vi "TEST_L0_SUM_(1ST)_NEW.vi"(7 "Serial Number":string="testFile", 8 "error in (no error)":errorcluster, 11 "Instrument VISA in":T1={"AWG VISA"="generadorpulsos", "Oscilloscope  VISA "="Oscilloscope", "Integration Board IP"="172.16.7.43", "connection ID"=refnum, "report out"=refnum, "report file path"=path "C:/Documents and Settings/CTA_LAB01/Desktop/L0_Asic/L0 Asic Test Data"}) -> (0 "error out":errorcluster, 3 "Instrument VISA out":T1={"AWG VISA"="generadorpulsos", "Oscilloscope  VISA "="Oscilloscope", "Integration Board IP"="172.16.7.43", "connection ID"=refnum, "report out"=refnum, "report file path"=path "C:/Documents and Settings/CTA_LAB01/Desktop/L0_Asic/L0 Asic Test Data"})   [LabVIEW 2009]
uses:
  <vilib>/Utility/NIReport.llb/NI_report.lvclass
  <vilib>/Utility/NIReport.llb/HTML/NI_HTML.lvclass
  Sum_Abrilader/L0_Sum_Adder Folder/C/Program Files/National Instruments/LabVIEW 2012/instr.lib/Agilent 8000 Series/Public/Configure/Configure Math (Binary Operation).vi
  <instrlib>/Agilent 8000 Series/Public/Data/Low Level/Fetch Measurement (More).vi
  <instrlib>/Agilent 8000 Series/Agilent 8000 Series.lvlib
panel:
  in  "Amp Scaler":dbl=1.1
  in  "Clip Select":i32[](array[numeric])=[1, 2, 3]
  in  "Atenuation":i32[](array[numeric])=[0, 15]
  in  "IB_Clip":i32[](array[numeric])=[7, 23, 31, 63]
  in  "Voltages":dbl[](array[numeric])=[0.05, 0.1, 0.2, 0.5, 0.8]
  in  "Channels":i32[](array[numeric])=[0, 1, 2, 3, 4, 5, 6]
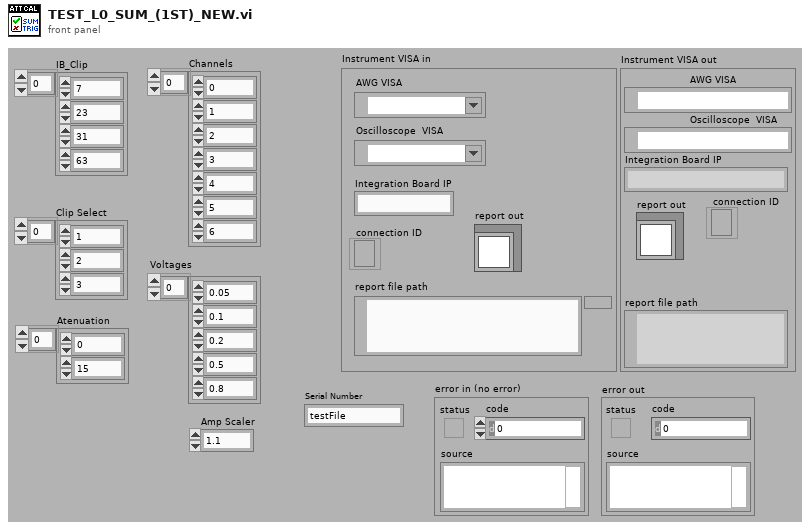
[diagram p1: front panel]
types:
  T1 = cluster{"AWG VISA":refnum<visa-resource-name>, "Oscilloscope  VISA ":refnum<visa-resource-name>, "Integration Board IP":string, "connection ID":refnum<k5>, "report out":refnum<class "NI_report.lvclass">, "report file path":path}
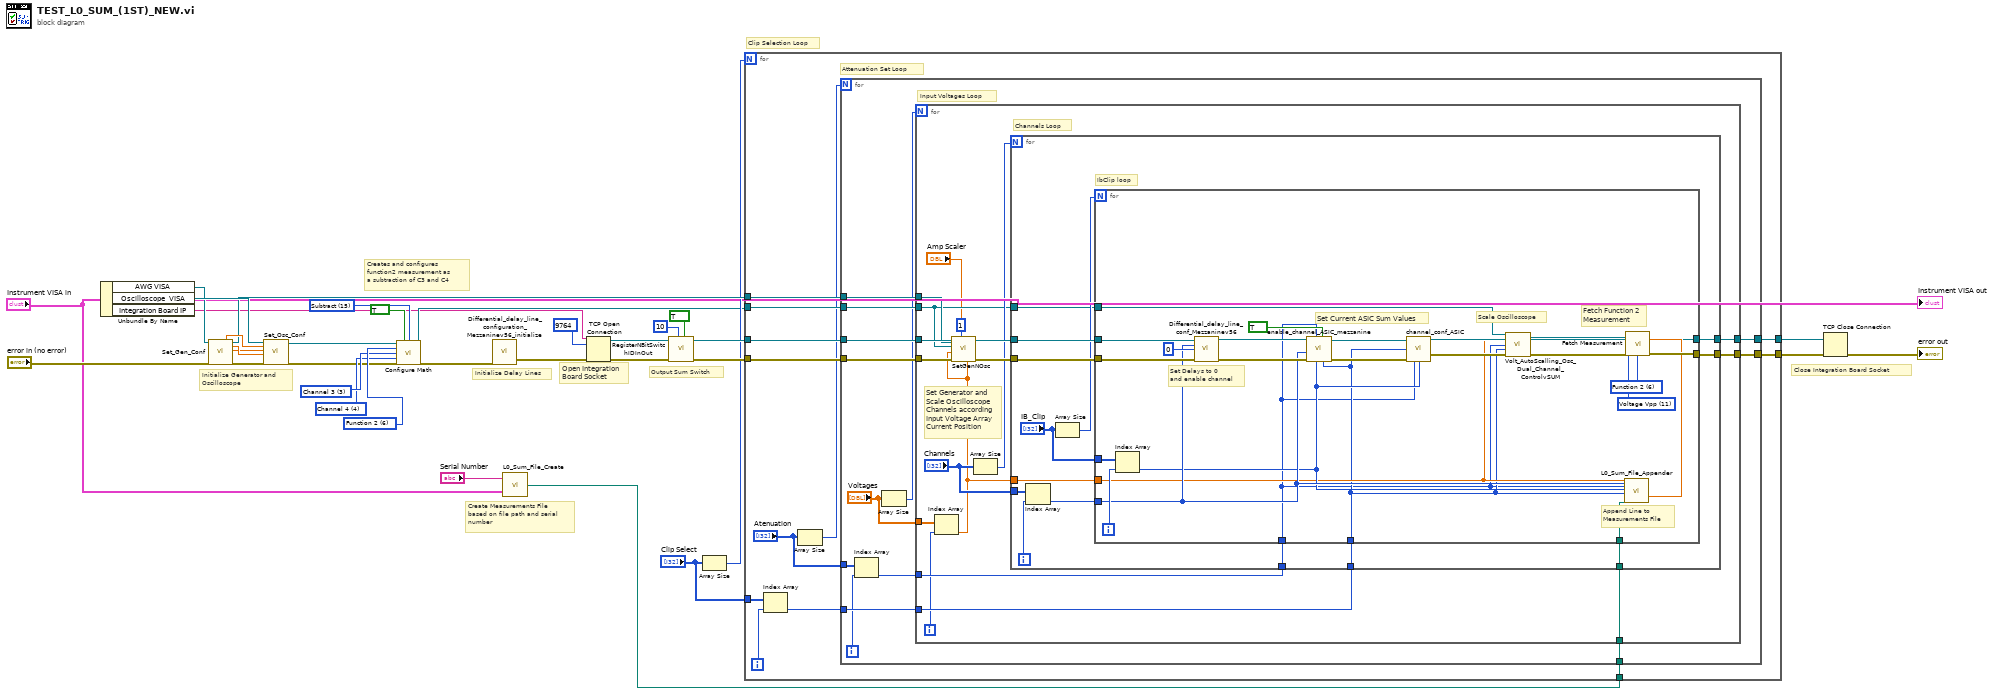
[diagram p0: block diagram]
diagram:
  w11 = u16 6 items=["Function 1"=5, "Function 2"=6, "Function 3"=7, "Function 4"=8] ("Math Channel (5: Function 1)")
  w12 = u16 15 items=["Add"=12, "Divide"=13, "Multiply"=14, "Subtract"=15, "Common Mode"=16, "Versus"=17] ("Math Operation (12: Add)")
  w10 = 3 items=["Channel 1"=1, "Channel 2"=2, "Channel 3"=3, "Channel 4"=4] ("Channel (1: Channel 1)")
  w9 = 4 items=["Channel 1"=1, "Channel 2"=2, "Channel 3"=3, "Channel 4"=4] ("Channel (1: Channel 1)")
  # "Clip Selection Loop"
  # "Create Measurements File\nbased on file path and serial\nnumber"
  # "Close Integration Board Socket"
  # "Output Sum Switch"
  # "Open Integration\nBoard Socket"
  # "Initialize Delay Lines"
  # "Initialize Generator and \nOscilloscope"
  # "Creates and configures\nfunction2 measurement as\na subtraction of C3 and C4"
  n1 = Unbundle By Name("Instrument VISA in") -> ("AWG VISA"=w30:refnum<visa-resource-name>, "Oscilloscope  VISA"=w31:refnum<visa-resource-name>, "Integration Board IP"=w4:string)
  n2 = call "Set_Gen_Conf.vi"("AWG VISA"=w30, "error in (no error)"="error in (no error)") -> ("Amplitude 1 OUT"=w28:dbl, "VISA resource name out"=w22:refnum<visa-resource-name>, "Pulse Width in seconds 1 OUT"=w27:dbl, "Trigger Level 1"=w26:dbl, "error out"=w32:errorcluster)  [unwired: 10 in, 3 out]
  n3 = call "Set_Osc_Conf.vi"("VISA resource name"=w31, "Amplitude IN"=w28, "Trigger Level IN"=w26, "Pulse Width in seconds IN"=w27, "error in (no error)"=w32) -> ("VISA resource name out"=w8:refnum<visa-resource-name>, "error out"=w7:errorcluster)  [unwired: 13 in]
  n4 = call-poly "Configure Math.vi"("VISA resource name"=w8, "Enable Math Channel (T:Enable)"=TRUE, "Math Operation (12: Add)"=w12, "Math Channel (5: Function 1)"=w11, "Math Operand (1: Channel 1)"=w10, "Math Operand (2: Channel 2)"=w9, "error in (no error)"=w7) -> ("VISA resource name out"=w5:refnum<visa-resource-name>, "error out"=w6:errorcluster)  [unwired: 7 in]
  n5 = call "Differential_delay_line_configuration_Mezzaninev56_initialize.vi"("error in (no error)"=w6) -> ("error out 2"=w25:errorcluster)  [unwired: 1 in]
  n6 = call "L0_Sum_File_Create.vi"("input cluster"="Instrument VISA in", "Serial Number"="Serial Number") -> ("appended path"=w1:path)
  n7 = TCP Open Connection(address=w4, remote port or service name=9764, error in (no error)=w25) -> (connection ID=w20:refnum<k5>, error out=w24:errorcluster)  [unwired: 2 in]
  n8 = call "RegisterNBitSwitchIDInOut.vi"("Switch Bit"=TRUE, "N Bit"=10, "error in (no error)"=w24, "connection ID"=w20) -> ("error out"=w21:errorcluster, "connection ID out"=w19:refnum<k5>)  [unwired: 5 in]
  n9 = Array Size(array="Clip Select") -> (size(s)=w16:i32)
  n10 = for {
    N: w16 -> [_]
    tunnel: w21 -> [w43]
    tunnel: [w44] -> w23
    tunnel: w19 -> [w46]
    tunnel: [w45] -> w14
    tunnel: w5 -> [w42]
    tunnel: w22 -> [w41]
    tunnel: "Clip Select" -> [w40]
    tunnel: w1 -> [w35]
    i -> [w39]
    # "Attenuation Set Loop"
    n11 = Index Array(array=w40, index=w39) -> (element=w38:i32)
    n12 = Array Size(array="Atenuation") -> (size(s)=w37:i32)
    n13 = for {
      N: w37 -> [_]
      tunnel: w46 -> [w59]
      tunnel: [w58] -> w45
      tunnel: [w57] -> w44
      tunnel: w43 -> [w56]
      tunnel: w42 -> [w55]
      tunnel: w41 -> [w54]
      tunnel: w38 -> [w53]
      tunnel: "Atenuation" -> [w52]
      tunnel: w35 -> [w47]
      i -> [w51]
      # "Input Voltages Loop"
      n14 = Index Array(array=w52, index=w51) -> (element=w50:i32)
      n15 = Array Size(array="Voltages") -> (size(s)=w49:i32)
      n16 = for {
        N: w49 -> [_]
        tunnel: w59 -> [w76]
        tunnel: [w75] -> w58
        tunnel: [w74] -> w57
        tunnel: w56 -> [w73]
        tunnel: w55 -> [w63]
        tunnel: w54 -> [w70]
        tunnel: w53 -> [w69]
        tunnel: w50 -> [w68]
        tunnel: "Voltages" -> [w67]
        tunnel: w47 -> [w62]
        i -> [w66]
        # "Channels Loop"
        # "Set Generator and\nScale Oscilloscope\nChannels according\nInput Voltage Array\nCurrent Position"
        n17 = Index Array(array=w67, index=w66) -> (element=w60:dbl)
        n18 = call "SetGenNOsc.vi"("Input Voltage"=w60, "Amp Scaler"="Amp Scaler", "NChannels"=1, "error in (no error)"=w73, "Output Voltage"=w60, "VISA resource name"=w63, "AWG VISA"=w70) -> ("error out 2"=w72:errorcluster)  [unwired: 4 in]
        n19 = Array Size(array="Channels") -> (size(s)=w65:i32)
        n20 = for {
          N: w65 -> [_]
          tunnel: w76 -> [w90]
          tunnel: [w89] -> w75
          tunnel: [w88] -> w74
          tunnel: w72 -> [w87]
          tunnel: w69 -> [w86]
          tunnel: w68 -> [w85]
          tunnel: "Channels" -> [w84]
          tunnel: w63 -> [w79]
          tunnel: w60 -> [w78]
          tunnel: w62 -> [w77]
          i -> [w83]
          # "IbClip loop"
          n21 = Index Array(array=w84, index=w83) -> (element=w82:i32)
          n22 = Array Size(array="IB_Clip") -> (size(s)=w81:i32)
          n23 = for {
            N: w81 -> [_]
            tunnel: w90 -> [w113]
            tunnel: [w98] -> w89
            tunnel: [w103] -> w88
            tunnel: w87 -> [w110]
            tunnel: w86 -> [w92]
            tunnel: w85 -> [w91]
            tunnel: w82 -> [w102]
            tunnel: "IB_Clip" -> [w107]
            tunnel: w79 -> [w95]
            tunnel: w78 -> [w93]
            tunnel: w77 -> [w99]
            i -> [w106]
            w105 = 11 items=["Rise Time", "Fall Time", "Frequency", "Period", "Voltage RMS(AC)", "Voltage RMS(DC)", "Voltage RMS (AC,cycle)", "Voltage RMS (DC,cycle)", "Voltage Max", "Voltage Min", "Voltage Middle", "Voltage Vpp", "Voltage High", "Voltage Low", "Voltage Average", "Voltage Average (cycle)", "Width Negative", "Width Positive", "Duty Cycle Positive", "Amplitude", "Overshoot", "Preshoot", "Voltage Base", "Voltage Upper", "Time Max", "Time Min", "Color Grade Crossing", "Color Grade Eye Width", "Color Grade Eye Height", "Color Grade Eye Q-Factory", "Color Grade Eye Duty Cycle Distortion(Percent)", "Color Grade Eye Duty Cycle Distortion(Time)", "Color Grade Eye Jitter(PP)", "Color Grade Eye Width(RMS)", "Cycle-cycle Duty Jitter(Rising)", "Cycle-cycle Duty Jitter(Falling)", "Cycle-cycle Jitter(Rising)", "Cycle-cycle Jitter(Falling)", "Cycle-cycle - Width", "Cycle-cycle + Width", "Date Rate", "Unit Interval", "FFT Delta Frequency", "FFT Delta Magnitude", "FFT Frequency", "FFT Magnitude", "Slew Rate", "Area (Entire Display)", "Area(Single Cycle)", "Duty Cycle (Rising)", "Duty Cycle (Falling)"] ("Measurement Function (0: Rise Time)")
            w104 = 6 items=["Channel 1"=1, "Channel 2"=2, "Channel 3"=3, "Channel 4"=4, "Function 1"=5, "Function 2"=6, "Function 3"=7, "Function 4"=8, "Memory 1"=9, "Memory 2"=10, "Memory 3"=11, "Memory 4"=12] ("Channel (1: Channel 1)")
            # "Scale Oscilloscope"
            # "Set Current ASIC Sum Values"
            # "Append Line to \nMeasurements File"
            # "Set Delays to 0 \nand enable channel"
            # "Fetch Function 2\nMeasurement"
            n24 = Index Array(array=w107, index=w106) -> (element=w101:i32)
            n25 = call "Differential_delay_line_conf_Mezzaninev56.vi"("connection ID"=w113, "channel"=w102, "Delay value"=u16 0, "error in (no error)"=w110) -> ("connection ID out"=w112:refnum<k5>, "error out 2"=w115:errorcluster)  [unwired: 4 in, 6 out]
            n26 = call "enable_channel_ASIC_mezzanine.vi"("Clip_sel_b"=w92, "maj/sum"=TRUE, "Ib_clipVb"=w101, "Att gain"=w91, "error in"=w115, "Channel"=w102, "connection ID"=w112) -> ("error out"=w114:errorcluster, "connection ID out"=w111:refnum<k5>)  [unwired: 2 in, 1 out]
            n27 = call "channel_conf_ASIC.vi"("connection ID"=w111, "Clip_sel_b"=w92, "error out"=w114, "Att gain"=w91, "Ib_ClipVb"=w101) -> ("connection ID out"=w98:refnum<k5>, "error out 2"=w97:errorcluster)  [unwired: 6 in, 3 out]
            n28 = call "Volt_AutoScalling_Osc_Dual_Channel_ControlvSUM.vi"("VISA Oscilloscope"=w95, "Voltage In"=w93, "Att"=w91, "Clip"=w92, "error in"=w97) -> ("VISA resource name out"=w94:refnum<visa-resource-name>, "error out"=w96:errorcluster)  [unwired: 9 in]
            n29 = call-poly <instrlib>:"Fetch Measurement.vi"("VISA resource name"=w94, "Channel (1: Channel 1)"=w104, "Measurement Function (0: Rise Time)"=w105, "error in (no error)"=w96) -> ("Measurement"=w100:dbl, "error out"=w103:errorcluster)  [unwired: 9 in, 1 out]
            n30 = call "L0_Sum_File_Appender.vi"("Vin"=w93, "CH"=w102, "Att"=w91, "IbClip"=w101, "Clip"=w92, "Vmeas"=w100, "file path (dialog if empty)"=w99) -> ()  [unwired: 21 in]
          }
        }
      }
    }
  }
  n31 = TCP Close Connection(connection ID=w14, error in (no error)=w23) -> (error out=→"error out":errorcluster)  [unwired: 1 in, 1 out]
  "Instrument VISA out" <- "Instrument VISA in"
